vi "main.vi"() -> ()   [LabVIEW 2019]
panel:
  out "Position":i32
  in  "OK":bool
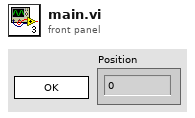
[diagram p1: front panel]
types:
  T1 = enum32{"Invalid", "Standard", "Closed", "Hidden", "Minimized", "Maximized"}
  T2 = enum32{"invalid app kind", "Development System", "Run Time System", "Student Edition", "Embedded LabVIEW", "Evaluation", "Custom"}
  T3 = cluster{"Core":cluster{"Current VI Reference":refnum<vi>, "Close Panel on Exit?":bool}, "Your Boolean data":bool, "Your string data":string}
  T4 = cluster{"Current VI Reference":refnum<vi>, "Close Panel on Exit?":bool}
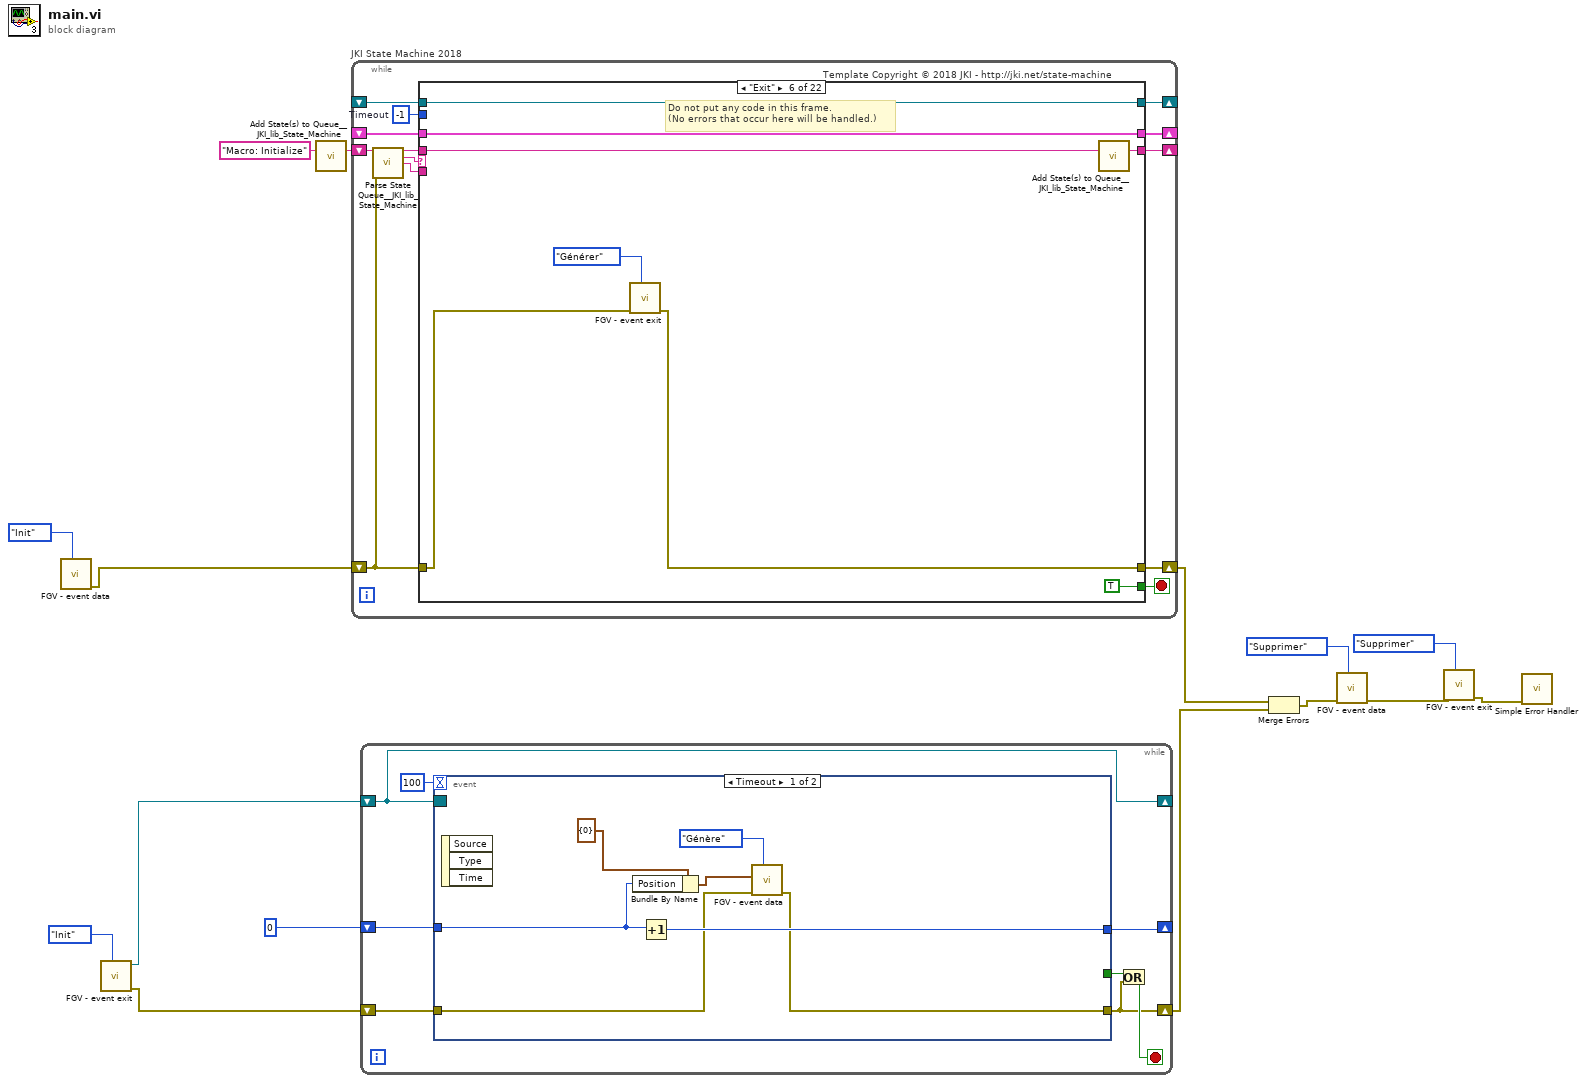
[diagram p0: block diagram]
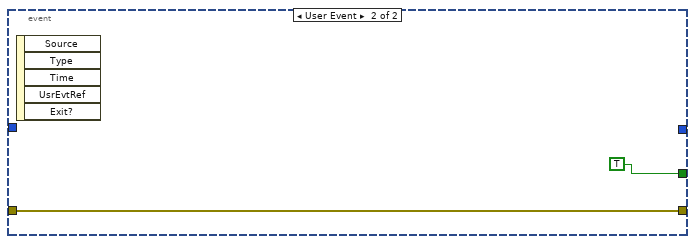
[diagram p2: hidden frame]
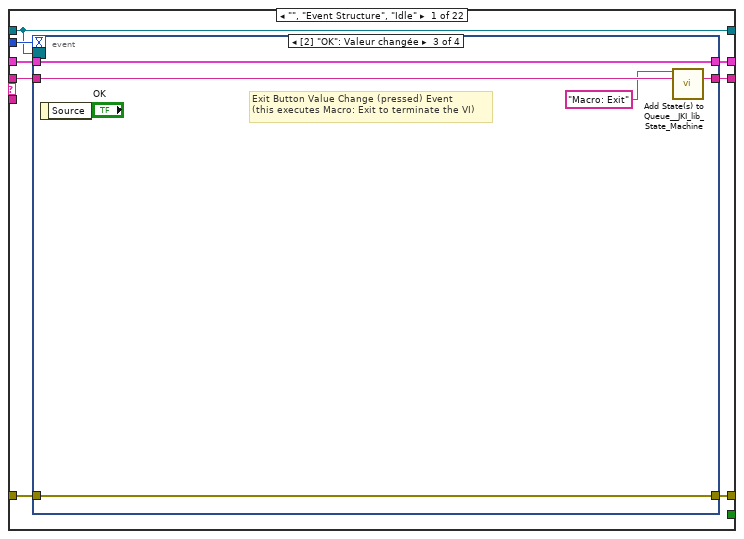
[diagram p3: hidden frame]
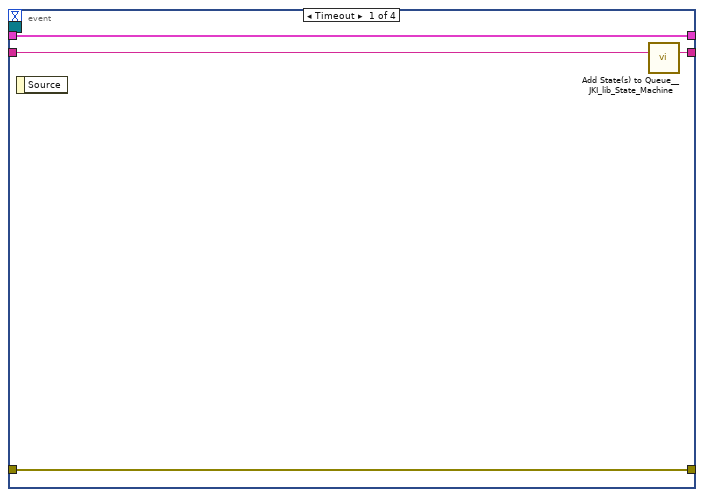
[diagram p4: hidden frame]
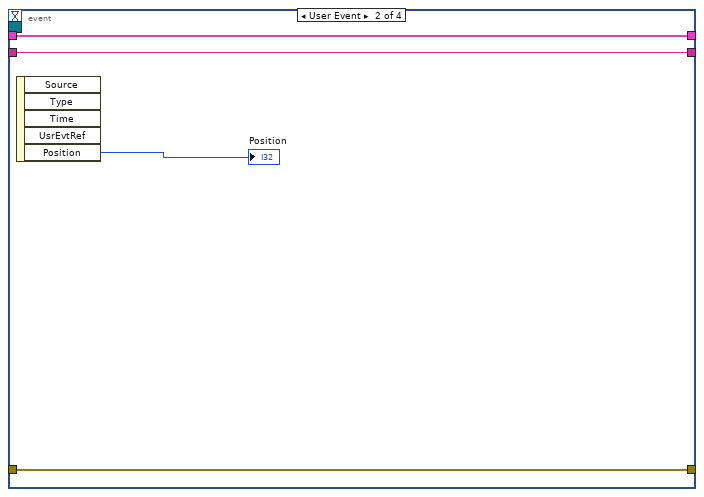
[diagram p5: hidden frame]
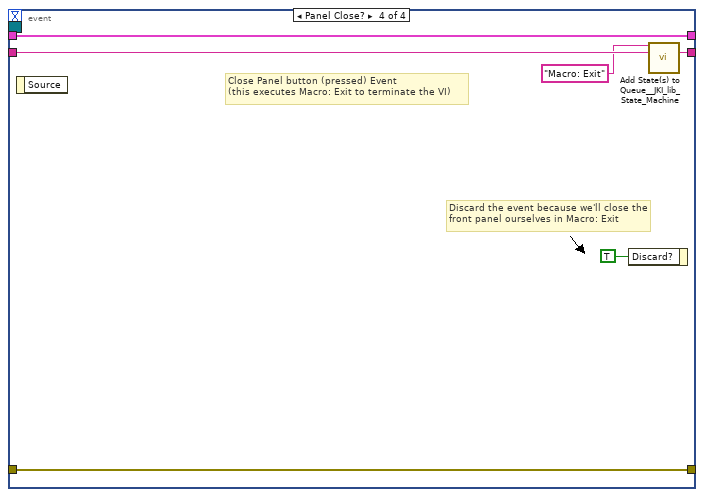
[diagram p6: hidden frame]
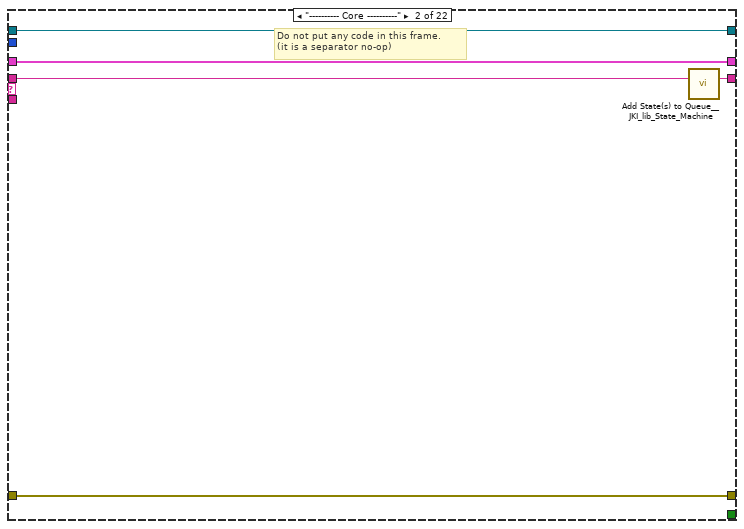
[diagram p7: hidden frame]
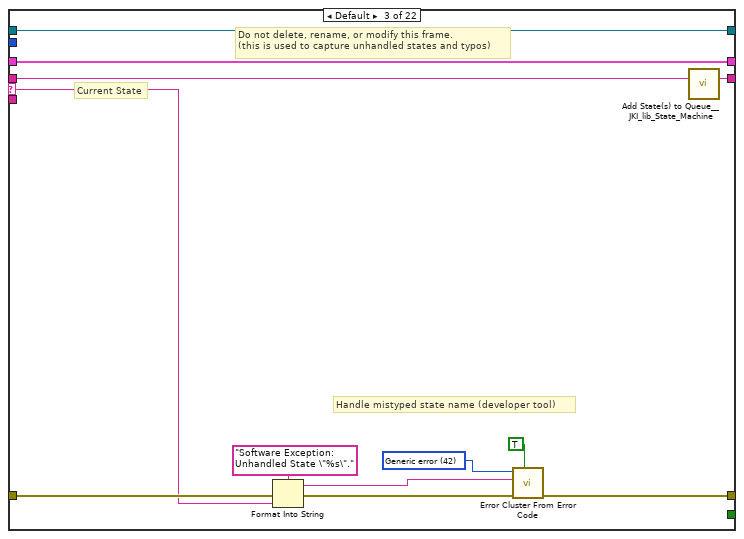
[diagram p8: hidden frame]
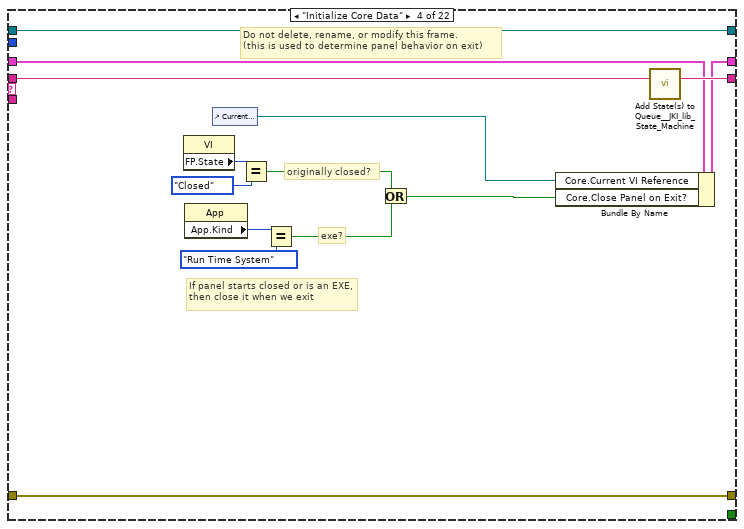
[diagram p9: hidden frame]
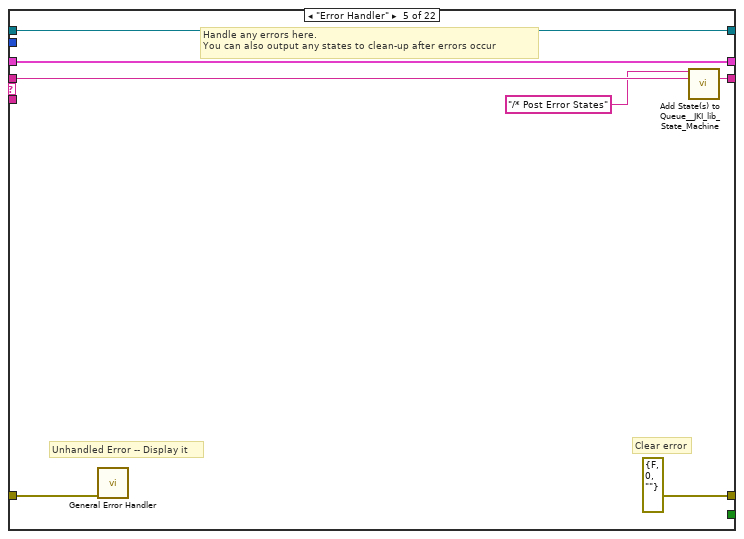
[diagram p10: hidden frame]
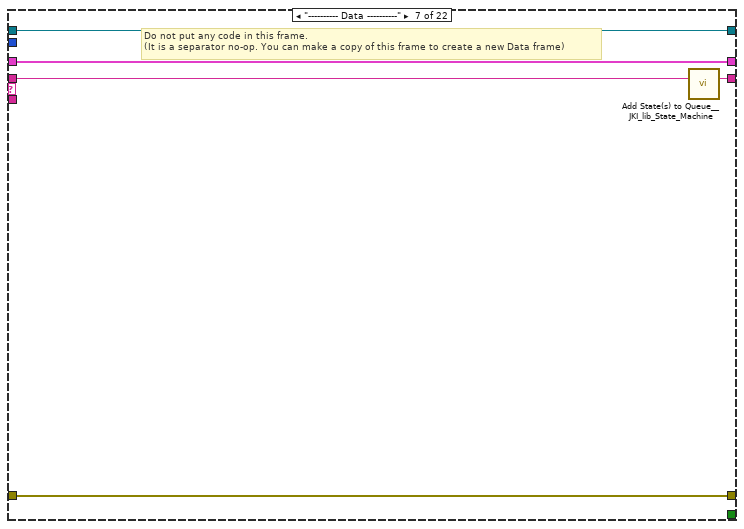
[diagram p11: hidden frame]
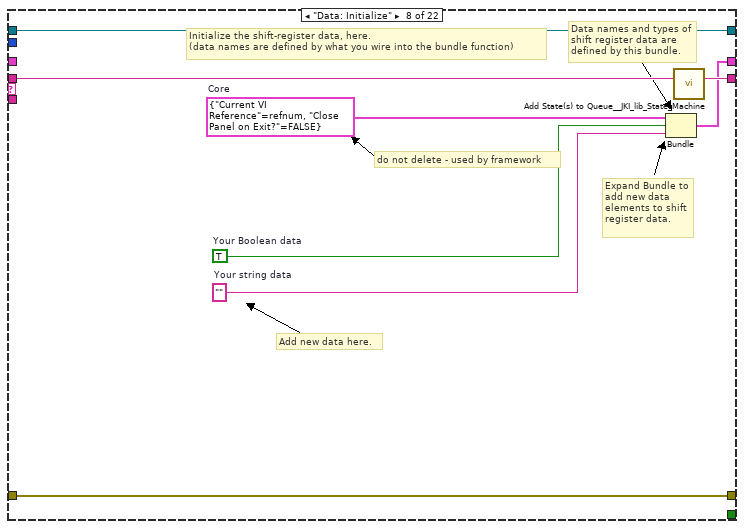
[diagram p12: hidden frame]
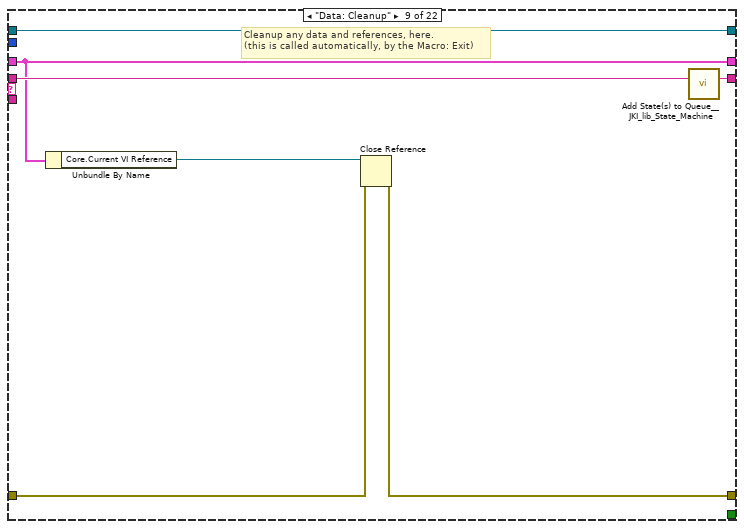
[diagram p13: hidden frame]
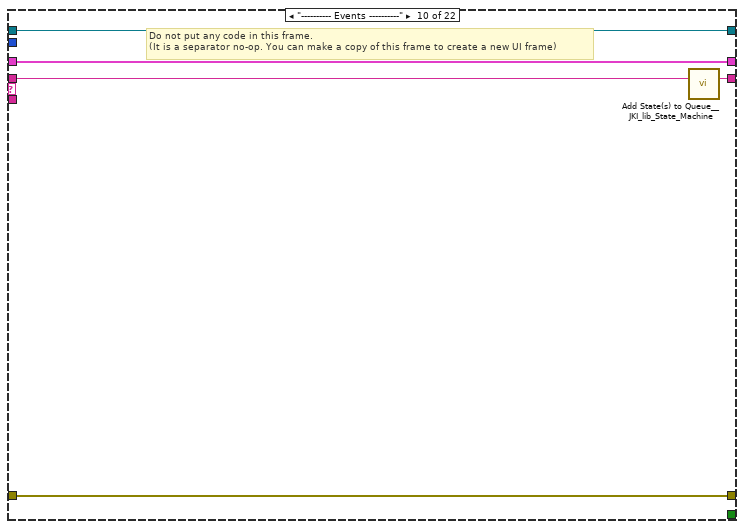
[diagram p14: hidden frame]
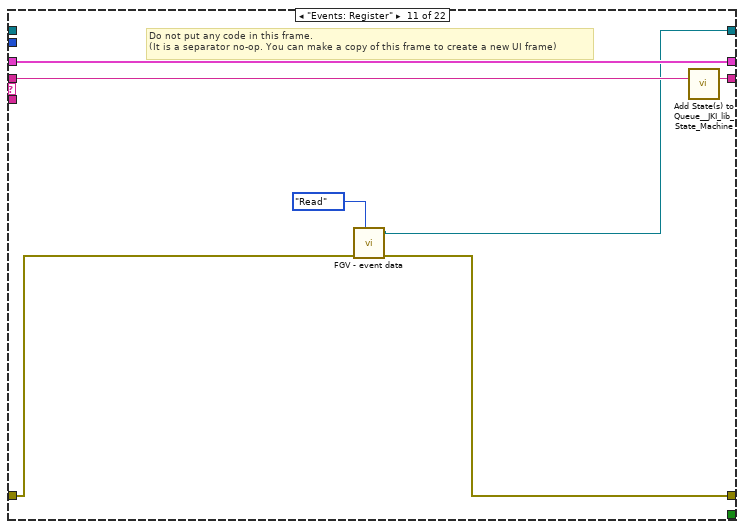
[diagram p15: hidden frame]
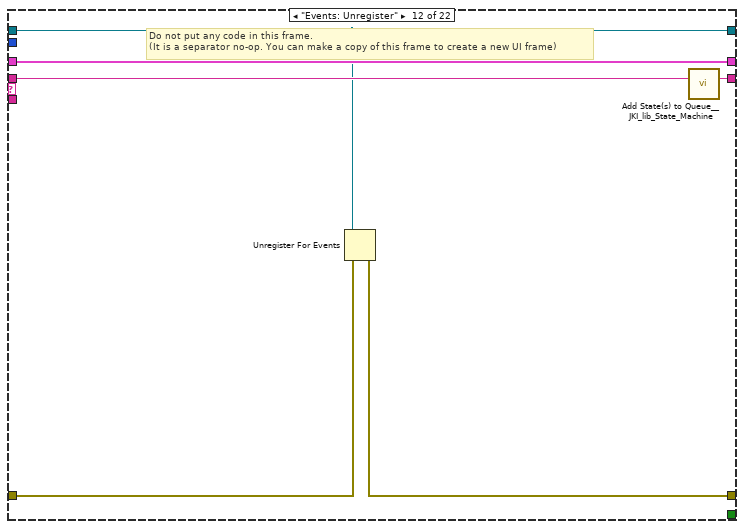
[diagram p16: hidden frame]
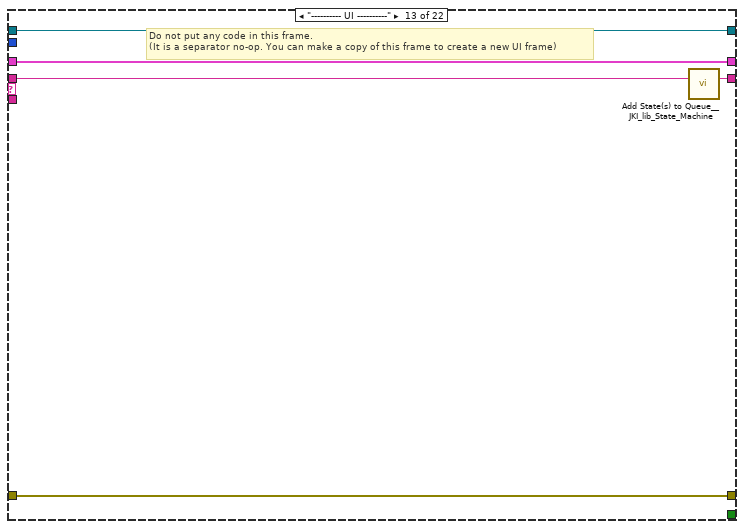
[diagram p17: hidden frame]
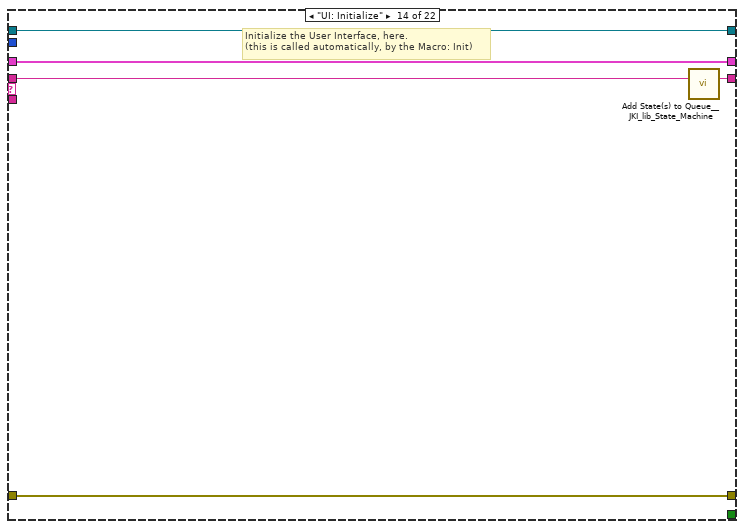
[diagram p18: hidden frame]
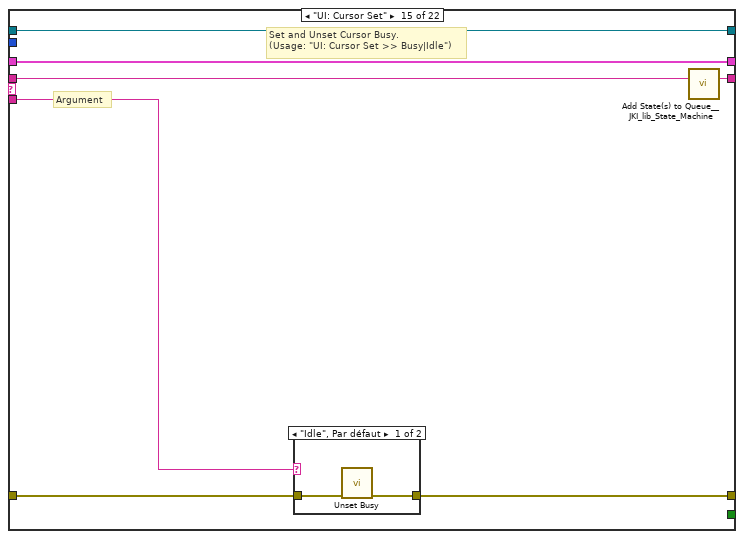
[diagram p19: hidden frame]
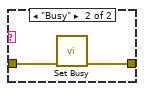
[diagram p20: hidden frame]
diagram:
  n1 = call "FGV - event data.vi"("Action (Read)"=enum16{"Init", "Read", "Génère", "Supprimer"}."Init") -> ("sortie d'erreur"=w13:errorcluster)  [unwired: 9 in, 1 out]
  n2 = call "FGV - event exit.vi"("Action (Read)"=enum16{"Init", "Read", "Générer", "Supprimer"}."Init") -> ("sortie d'erreur"=w6:errorcluster, "Refnum d'abonnement à des événements"=w11:refnum<event-registration>)  [unwired: 9 in]
  n3 = call <vilib>:"Add State(s) to Queue__JKI_lib_State_Machine.vi"("State(s) in (\"\")"="Macro: Initialize") -> ("States Out"=w15:string)  [unwired: 14 in]
  n4 = while "JKI State Machine 2018" {
    shift-right: [w21] -> _
    shift-left: _ -> [w20]
    shift-right: [w24] -> w9
    shift-left: w13 -> [w18]
    shift-right: [w23] -> _
    shift-left: w15 -> [w25]
    shift-right: [w17] -> _
    shift-left: _ -> [w16]
    stop <- w22 stop-if-true
    w19 = -1  # Timeout
    # "Template Copyright © 2018 JKI - http://jki.net/state-machine"
    n5 = call <vilib>:"Parse State Queue__JKI_lib_State_Machine.vi"("State Queue"=w25, "Error In (no error)"=w18) -> ("Remaining States"=w27:string, "Current State"=w28:string, "Arguments"=w26:string)  [unwired: 11 in]
    n6 = case shown="\"Exit\"" w28 {
      selector: w28 -> [_ _ w62 _ _ _ _ _ _ _ _ _ _ _ _ _ _ _ _ _ _ _]
      tunnel: w27 -> [w36 w60 w66 w86 w93 w101 w106 w114 w121 w126 w133 w139 w144 w149 w156 w168 w238 w244 w255 w260 w265 w270]
      tunnel: w26 -> [_ _ _ _ _ _ _ _ _ _ _ _ _ _ w151 w162 _ _ _ _ _ _]
      tunnel: w20 -> [w34 w57 w64 w79 w90 w99 w103 _ w116 w123 w131 w137 w141 w147 w154 w164 w235 w241 w252 w257 w262 w267]
      tunnel: [w33 w58 w68 w83 errorcluster {"status"=FALSE, "code"=0, "source"=""} ("error out") w95 w104 w111 w117 w124 w128 w134 w142 w146 w152 w165 w236 w242 w253 w258 w263 w268] -> w24
      tunnel: w18 -> [w32 w58 w67 w83 w89 w96 w104 w111 w118 w124 w129 w135 w142 w146 w153 w166 w236 w242 w253 w258 w263 w268]
      tunnel: [w35 w59 w65 w85 w92 w100 w105 w113 w120 w125 w132 w138 w143 w148 w155 w167 w237 w243 w254 w259 w264 w269] -> w23
      tunnel: [_ _ _ _ _ TRUE _ _ _ _ _ _ _ _ _ _ _ _ _ _ _ _] -> w22
      tunnel: [w31 w57 w64 w84 w90 w99 w103 w112 w116 w123 w131 w137 w141 w147 w154 w164 w235 w241 w252 w257 w262 w267] -> w21
      tunnel: w19 -> [w30 _ _ _ _ _ _ _ _ _ _ _ _ _ _ _ _ _ _ _ _ _]
      tunnel: [w29 w56 w61 w73 w87 w97 w102 w107 w115 w122 w130 w136 w140 w145 w150 w161 w234 w239 w245 w256 w261 w266] -> w17
      tunnel: w16 -> [w29 w56 w61 w73 w87 w97 w102 w107 w115 w122 _ w136 w140 w145 w150 w161 w234 w239 w245 w256 w261 w266]
      frame "", "Event Structure", "Idle" {
        n7 = event shown="[2] \"OK\": Valeur changée" {
          selector: w29 -> [_ _ _ _]
          dyn-events: _ -> [_ _ _ _]
          timeout: w30 -> [_ _ _ _]
          tunnel: w36 -> [w40 w42 w49 w55]
          tunnel: [w39 w42 w48 w54] -> w35
          tunnel: w34 -> [w37 w43 w46 w52]
          tunnel: [w38 w41 w47 w53] -> w33
          tunnel: w32 -> [w38 w41 w47 w53]
          tunnel: [w37 w43 w46 w52] -> w31
          event Timeout {
            n8 = event-data() -> ()  [unwired: 1 in, 1 out]
            n9 = call <vilib>:"Add State(s) to Queue__JKI_lib_State_Machine.vi"("State(s) in (\"\")"=w40) -> ("States Out"=w39:string)  [unwired: 14 in]
          }
          event User Event {
            n10 = event-data() -> ("Position"=→"Position":i32)  [unwired: 1 in, 4 out]
          }
          event "OK": Value Change {
            # "Exit Button Value Change (pressed) Event\n(this executes Macro: Exit to terminate the VI)"
            n11 = event-data() -> ()  [unwired: 1 in, 1 out]
            n12 = call <vilib>:"Add State(s) to Queue__JKI_lib_State_Machine.vi"("State(s) in Front (\"\")"="Macro: Exit", "State(s) in (\"\")"=w49) -> ("States Out"=w48:string)  [unwired: 13 in]
          }
          event Panel Close? {
            # "Discard the event because we'll close the front panel ourselves in Macro: Exit"
            # "Close Panel button (pressed) Event\n(this executes Macro: Exit to terminate the VI)"
            n13 = event-data() -> ()  [unwired: 1 in, 1 out]
            n14 = event-data("Discard?"=TRUE) -> ()  [unwired: 1 in, 1 out]
            n15 = call <vilib>:"Add State(s) to Queue__JKI_lib_State_Machine.vi"("State(s) in Front (\"\")"="Macro: Exit", "State(s) in (\"\")"=w55) -> ("States Out"=w54:string)  [unwired: 13 in]
          }
        }
      }
      frame "---------- Core ----------" {
        # "Do not put any code in this frame.\n(it is a separator no-op)"
        n16 = call <vilib>:"Add State(s) to Queue__JKI_lib_State_Machine.vi"("State(s) in (\"\")"=w60) -> ("States Out"=w59:string)  [unwired: 14 in]
      }
      frame Default {
        w71 = 42 items=["No error", "Argument error", "Memory is full", "Out of zone", "End of file", "File already open", "Generic file I/O error", "File not found", "File permission error", "Disk is full", "Duplicate path", "Too many files open", "System feature not enabled", "Resource file not found", "Cannot add resource", "Resource not found", "Image not found", "Image memory error", "Pen does not exist", "Config type invalid", "Config token not found", "Config parse error", "Config memory error", "Bad external code format", "Bad external code offset", "External code not present", "Null window", "Destroy window error", "Null menu", "Print aborted", "Bad print record", "Print driver error", "Windows error during printing", "Memory error during printing", "Print dialog error", "Generic print error", "Invalid device refnum", "Device not found", "Device parameter error", "Device unit error", "Cannot open device", "Device call aborted", "Generic error", "Cancelled by user", "Object ID too low", "Object ID too high", "Object not in heap", "Unknown heap", "Unknown object (invalid DefProc)", "Unknown object (DefProc not in table)", "Message out of range", "Invalid (null) method", "Unknown message", "Manager call not supported", "Bad address", "Network operation in progress", "Network operation timed out", "Connection is busy", "Network attribute not supported", "Network error", "Address in use", "System out of memory", "Connection aborted", "Connection refused", "Not connected", "Already connected", "Connection closed", "Initialization error (interapplication manager)", "Bad occurrence", "Wait on unbound occurrence handler", "Occurrence queue overflow", "Datalog type conflict", "Unused", "Unrecognized type (interapplication manager)", "Memory corrupt", "Failed to make temporary DLL", "Old CIN version", "Drag socket not found", "Failed to load drop-object", "Failed to register OLE object", "Failed to release OLE object", "Format specifier type mismatch", "Unknown format specifier", "Too few format specifiers", "Too many format specifiers", "Scan failed", "Newer CIN version", "Error converting to variant", "Runtime menu error", "Password tampered", "Variant attribute not found", "Incompatible variant data type", "Event data is not available", "Event Store is not present", "Occurrence is not found", "Event Queue is not created", "Event info is not available", "Refnum passed is NULL", "Error retrieving Class GUID", "Error retrieving CoClass GUID", "Error retrieving TypeLib GUID.", "Bad built application magic bytes.", "Specific driver is different from the specific driver associated with the Logical Name.", "There is no session opened to the class driver.", "Max Error", "MAX - Error with config objects", "MAX - Error loading configuration", "MAX - Group not supported"]
        # "Current State"
        # "Do not delete, rename, or modify this frame.\n(this is used to capture unhandled states and typos)"
        # "Handle mistyped state name (developer tool)"
        n17 = Format Into String(format string="Software Exception: Unhandled State \"%s\"." ("message"), error in=w67, w62) -> (resulting string=w70:string, error out=w69:errorcluster)  [unwired: 1 in]
        n18 = call <vilib>:"Error Cluster From Error Code.vi"("show call chain? (False)"=TRUE, "error in (no error)"=w69, "error message (\"\")"=w70, "error code (0)"=w71) -> ("error out"=w68:errorcluster)  [unwired: 5 in]
        n19 = call <vilib>:"Add State(s) to Queue__JKI_lib_State_Machine.vi"("State(s) in (\"\")"=w66) -> ("States Out"=w65:string)  [unwired: 14 in]
      }
      frame "Initialize Core Data" {
        # "Do not delete, rename, or modify this frame.\n(this is used to determine panel behavior on exit)"
        # "originally closed?"
        # "exe?"
        # "If panel starts closed or is an EXE, then close it when we exit"
        n20 = property class="VI"() -> ("FP.State"=w76:T1)  [unwired: 2 in, 2 out]
        n21 = property class="App"() -> ("App.Kind"=w82:T2)  [unwired: 2 in, 2 out]
        n22 = control-ref of="Current VI Reference"() -> (w77:refnum<vi>)
        n23 = Equal?(x=w76, y=T1."Closed" ("Front Panel Window:State")) -> (x = y?=w74:bool)
        n24 = Equal?(x=w82, y=T2."Run Time System" ("Application:Kind")) -> (x = y?=w80:bool)
        n25 = Or(x=w74, y=w80) -> (x .or. y?=w78:bool)
        n26 = Bundle By Name(cluster=w79, "Core.Current VI Reference"=w77, "Core.Close Panel on Exit?"=w78) -> (w84:T3)
        n27 = call <vilib>:"Add State(s) to Queue__JKI_lib_State_Machine.vi"("State(s) in (\"\")"=w86) -> ("States Out"=w85:string)  [unwired: 14 in]
      }
      frame "Error Handler" {
        # "Unhandled Error -- Display it"
        # "Handle any errors here.\nYou can also output any states to clean-up after errors occur"
        # "Clear error"
        n28 = call <vilib>:"General Error Handler.vi"("error in (no error)"=w89) -> ()  [unwired: 10 in, 5 out]
        n29 = call <vilib>:"Add State(s) to Queue__JKI_lib_State_Machine.vi"("State(s) in Front (\"\")"="/* Post Error States", "State(s) in (\"\")"=w93) -> ("States Out"=w92:string)  [unwired: 13 in]
      }
      frame "Exit" {
        # "Do not put any code in this frame.\n(No errors that occur here will be handled.)"
        n30 = call "FGV - event exit.vi"("Action (Read)"=enum16{"Init", "Read", "Générer", "Supprimer"}."Générer", "entrée d'erreur (pas d'erreur)"=w96) -> ("sortie d'erreur"=w95:errorcluster)  [unwired: 8 in, 1 out]
        n31 = call <vilib>:"Add State(s) to Queue__JKI_lib_State_Machine.vi"("State(s) in (\"\")"=w101) -> ("States Out"=w100:string)  [unwired: 14 in]
      }
      frame "---------- Data ----------" {
        # "Do not put any code in this frame.\n(It is a separator no-op. You can make a copy of this frame to create a new Data frame)"
        n32 = call <vilib>:"Add State(s) to Queue__JKI_lib_State_Machine.vi"("State(s) in (\"\")"=w106) -> ("States Out"=w105:string)  [unwired: 14 in]
      }
      frame "Data: Initialize" {
        w108 = T4 {"Current VI Reference"=refnum, "Close Panel on Exit?"=FALSE}  # Core
        w110 = TRUE  # Your Boolean data
        w109 = ""  # Your string data
        # "do not delete - used by framework"
        # "Expand Bundle to add new data elements to shift register data."
        # "Add new data here."
        # "Data names and types of shift register data are defined by this bundle."
        # "Initialize the shift-register data, here.\n(data names are defined by what you wire into the bundle function)"
        n33 = Bundle("Core"=w108, "Your Boolean data"=w110, "Your string data"=w109) -> (w112:T3)  [unwired: 1 in]
        n34 = call <vilib>:"Add State(s) to Queue__JKI_lib_State_Machine.vi"("State(s) in (\"\")"=w114) -> ("States Out"=w113:string)  [unwired: 14 in]
      }
      frame "Data: Cleanup" {
        # "Cleanup any data and references, here.\n(this is called automatically, by the Macro: Exit)"
        n35 = Unbundle By Name(w116) -> ("Core.Current VI Reference"=w119:refnum<vi>)
        n36 = Close Reference(reference=w119, error in (no error)=w118) -> (error out=w117:errorcluster)
        n37 = call <vilib>:"Add State(s) to Queue__JKI_lib_State_Machine.vi"("State(s) in (\"\")"=w121) -> ("States Out"=w120:string)  [unwired: 14 in]
      }
      frame "---------- Events ----------" {
        # "Do not put any code in this frame.\n(It is a separator no-op. You can make a copy of this frame to create a new UI frame)"
        n38 = call <vilib>:"Add State(s) to Queue__JKI_lib_State_Machine.vi"("State(s) in (\"\")"=w126) -> ("States Out"=w125:string)  [unwired: 14 in]
      }
      frame "Events: Register" {
        # "Do not put any code in this frame.\n(It is a separator no-op. You can make a copy of this frame to create a new UI frame)"
        n39 = call "FGV - event data.vi"("Action (Read)"=enum16{"Init", "Read", "Génère", "Supprimer"}."Read", "entrée d'erreur (pas d'erreur)"=w129) -> ("sortie d'erreur"=w128:errorcluster, "Refnum d'abonnement à des événements"=w130:refnum<event-registration>)  [unwired: 8 in]
        n40 = call <vilib>:"Add State(s) to Queue__JKI_lib_State_Machine.vi"("State(s) in (\"\")"=w133) -> ("States Out"=w132:string)  [unwired: 14 in]
      }
      frame "Events: Unregister" {
        # "Do not put any code in this frame.\n(It is a separator no-op. You can make a copy of this frame to create a new UI frame)"
        n41 = Unregister For Events(event registration refnum=w136, error in=w135) -> (error out=w134:errorcluster)
        n42 = call <vilib>:"Add State(s) to Queue__JKI_lib_State_Machine.vi"("State(s) in (\"\")"=w139) -> ("States Out"=w138:string)  [unwired: 14 in]
      }
      frame "---------- UI ----------" {
        # "Do not put any code in this frame.\n(It is a separator no-op. You can make a copy of this frame to create a new UI frame)"
        n43 = call <vilib>:"Add State(s) to Queue__JKI_lib_State_Machine.vi"("State(s) in (\"\")"=w144) -> ("States Out"=w143:string)  [unwired: 14 in]
      }
      frame "UI: Initialize" {
        # "Initialize the User Interface, here.\n(this is called automatically, by the Macro: Init)"
        n44 = call <vilib>:"Add State(s) to Queue__JKI_lib_State_Machine.vi"("State(s) in (\"\")"=w149) -> ("States Out"=w148:string)  [unwired: 14 in]
      }
      frame "UI: Cursor Set" {
        # "Argument"
        # "Set and Unset Cursor Busy.\n(Usage: \"UI: Cursor Set >> Busy|Idle\")"
        n45 = case shown="\"Idle\", Par défaut" w151 {
          tunnel: w153 -> [w158 w160]
          tunnel: [w157 w159] -> w152
          frame "Idle", Default {
            n46 = call <vilib>:"Unset Busy.vi"("error in (no error)"=w158) -> ("error out"=w157:errorcluster)  [unwired: 10 in]
          }
          frame "Busy" {
            n47 = call <vilib>:"Set Busy.vi"("error in (no error)"=w160) -> ("error out"=w159:errorcluster)  [unwired: 9 in, 1 out]
          }
        }
        n48 = call <vilib>:"Add State(s) to Queue__JKI_lib_State_Machine.vi"("State(s) in (\"\")"=w156) -> ("States Out"=w155:string)  [unwired: 14 in]
      }
      frame "UI: Front Panel State" {
        # "Argument"
        # "Set Front Panel Open or Closed\n(Usage: \"UI: Front Panel State >> Open|Close\")"
        n49 = Unbundle By Name(w164) -> ("Core.Current VI Reference"=w163:refnum<vi>)
        n50 = case shown="\"Minimize\", \"Minimized\"" w162 {
          tunnel: w166 -> [w174 w189 w200 w213 w226]
          tunnel: [w176 w190 w202 w215 w228] -> w165
          tunnel: w163 -> [w175 w187 w201 w214 w227]
          frame "Open", "Standard", Default {
            w169 = T1."Standard" ("State")
            n51 = property class="VI"(reference=w175, error in=w174) -> (reference out=w172:refnum<vi>, error out=w173:errorcluster, "FP.State"=w171:T1)
            n52 = Not Equal?(x=w171, y=w169) -> (x != y?=w170:bool)
            n53 = case shown="Vrai" w170 {
              tunnel: [w180 w182] -> w176
              tunnel: w173 -> [w179 w182]
              tunnel: w172 -> [w178 _]
              tunnel: w169 -> [w177 _]
              frame True {
                n54 = invoke class="VI" method="FA.Ouvrir"(reference=w178, error in=w179, "Activate"=TRUE, "State"=w177) -> (error out=w180:errorcluster)  [unwired: 1 in, 4 out]
              }
              frame False {
              }
            }
          }
          frame "Close", "Closed" {
            n55 = property class="VI"(reference=w187, error in=w189) -> (reference out=w186:refnum<vi>, error out=w188:errorcluster, "FP.State"=w184:T1)
            n56 = Not Equal?(x=w184, y=T1."Closed" ("Front Panel Window:State")) -> (x != y?=w183:bool)
            n57 = case shown="Vrai" w183 {
              tunnel: [w191 w194] -> w190
              tunnel: w188 -> [w191 w193]
              tunnel: w186 -> [_ w192]
              frame False {
              }
              frame True {
                n58 = invoke class="VI" method="FA.Fermer"(reference=w192, error in=w193) -> (error out=w194:errorcluster)  [unwired: 1 in, 2 out]
              }
            }
          }
          frame "Hidden", "Hide" {
            w195 = T1."Hidden" ("State")
            n59 = property class="VI"(reference=w201, error in=w200) -> (reference out=w198:refnum<vi>, error out=w199:errorcluster, "FP.State"=w197:T1)
            n60 = Not Equal?(x=w197, y=w195) -> (x != y?=w196:bool)
            n61 = case shown="Vrai" w196 {
              tunnel: [w206 w207] -> w202
              tunnel: w199 -> [w205 w207]
              tunnel: w198 -> [w204 _]
              tunnel: w195 -> [w203 _]
              frame True {
                n62 = invoke class="VI" method="FA.Ouvrir"(reference=w204, error in=w205, "State"=w203) -> (error out=w206:errorcluster)  [unwired: 2 in, 4 out]
              }
              frame False {
              }
            }
          }
          frame "Minimize", "Minimized" {
            w208 = T1."Minimized" ("State")
            n63 = property class="VI"(reference=w214, error in=w213) -> (reference out=w211:refnum<vi>, error out=w212:errorcluster, "FP.State"=w210:T1)
            n64 = Not Equal?(x=w210, y=w208) -> (x != y?=w209:bool)
            n65 = case shown="Vrai" w209 {
              tunnel: [w219 w220] -> w215
              tunnel: w212 -> [w218 w220]
              tunnel: w211 -> [w217 _]
              tunnel: w208 -> [w216 _]
              frame True {
                n66 = invoke class="VI" method="FA.Ouvrir"(reference=w217, error in=w218, "State"=w216) -> (error out=w219:errorcluster)  [unwired: 2 in, 4 out]
              }
              frame False {
              }
            }
          }
          frame "Maximize", "Maximized" {
            w221 = T1."Maximized" ("State")
            n67 = property class="VI"(reference=w227, error in=w226) -> (reference out=w224:refnum<vi>, error out=w225:errorcluster, "FP.State"=w223:T1)
            n68 = Not Equal?(x=w223, y=w221) -> (x != y?=w222:bool)
            n69 = case shown="Vrai" w222 {
              tunnel: [w232 w233] -> w228
              tunnel: w225 -> [w231 w233]
              tunnel: w224 -> [w230 _]
              tunnel: w221 -> [w229 _]
              frame True {
                n70 = invoke class="VI" method="FA.Ouvrir"(reference=w230, error in=w231, "State"=w229) -> (error out=w232:errorcluster)  [unwired: 2 in, 4 out]
              }
              frame False {
              }
            }
          }
        }
        n71 = call <vilib>:"Add State(s) to Queue__JKI_lib_State_Machine.vi"("State(s) in (\"\")"=w168) -> ("States Out"=w167:string)  [unwired: 14 in]
      }
      frame "---------- Macro ----------" {
        # "Do not put any code in this frame.\n(It is a separator no-op. You can make a copy of this frame to create a new Macro frame)"
        n72 = call <vilib>:"Add State(s) to Queue__JKI_lib_State_Machine.vi"("State(s) in (\"\")"=w238) -> ("States Out"=w237:string)  [unwired: 14 in]
      }
      frame "Macro: Initialize" {
        # "Initialization Macro\n(This is called once, when the VI starts)"
        n73 = call <vilib>:"Add State(s) to Queue__JKI_lib_State_Machine.vi"("State(s) in Front (\"\")"="Data: Initialize\nInitialize Core Data\nEvents: Register\nUI: Initialize\nUI: Front Panel State >> Open", "State(s) in (\"\")"=w244) -> ("States Out"=w243:string)  [unwired: 13 in]
      }
      frame "Macro: Exit" {
        # "Exit Macro\n(This is called once, when the VI exits)"
        n74 = Unbundle By Name(w252) -> ("Core.Close Panel on Exit?"=w251:bool)
        n75 = Select(t="UI: Front Panel State >> Close", s=w251, f="") -> (s? t:f=w248:string)
        n76 = call <vilib>:"Add State(s) to Queue__JKI_lib_State_Machine.vi"("State(s) in (\"\")"=w248, "State(s) at Back (\"\")"="Data: Cleanup\nEvents: Unregister\nExit") -> ("States Out"=w246:string)  [unwired: 13 in]
        n77 = call <vilib>:"Add State(s) to Queue__JKI_lib_State_Machine.vi"("State(s) in Front (\"\")"=w246, "State(s) in (\"\")"=w255) -> ("States Out"=w254:string)  [unwired: 13 in]
      }
      frame "---------- New Category ----------" {
        # "Template Separator\n(You can make a copy of, or modify, this frame)"
        n78 = call <vilib>:"Add State(s) to Queue__JKI_lib_State_Machine.vi"("State(s) in (\"\")"=w260) -> ("States Out"=w259:string)  [unwired: 14 in]
      }
      frame "New Category: 1" {
        # "Your code here.\n(You can make a copy of, or modify, this frame)"
        n79 = call <vilib>:"Add State(s) to Queue__JKI_lib_State_Machine.vi"("State(s) in (\"\")"=w265) -> ("States Out"=w264:string)  [unwired: 14 in]
      }
      frame "New Category: 2" {
        # "Your code here.\n(You can make a copy of, or modify, this frame)"
        n80 = call <vilib>:"Add State(s) to Queue__JKI_lib_State_Machine.vi"("State(s) in (\"\")"=w270) -> ("States Out"=w269:string)  [unwired: 14 in]
      }
    }
  }
  n81 = while {
    shift-right: [w276] -> _
    shift-left: 0 -> [w277]
    shift-right: [w274] -> _
    shift-left: w11 -> [w274]
    shift-right: [w271] -> w5
    shift-left: w6 -> [w272]
    stop <- w275 stop-if-true
    n82 = event shown="[0] Timeout" {
      selector: w274 -> [_ _]
      dyn-events: _ -> [_ _]
      timeout: 100 -> [_ _]
      tunnel: w277 -> [w284 _]
      tunnel: [w285 _] -> w276
      tunnel: [_ TRUE] -> w273
      tunnel: [w280 w286] -> w271
      tunnel: w272 -> [w279 w286]
      event Timeout {
        n83 = event-data() -> ()  [unwired: 1 in, 3 out]
        n84 = Bundle By Name(cluster=cluster{"Position":i32} {"Position"=0} ("données d'événement"), "Position"=w284) -> (w281:cluster{"Position":i32})
        n85 = Increment(x=w284) -> (x+1=w285:i32)
        n86 = call "FGV - event data.vi"("Action (Read)"=enum16{"Init", "Read", "Génère", "Supprimer"}."Génère", "entrée d'erreur (pas d'erreur)"=w279, "Event Data"=w281) -> ("sortie d'erreur"=w280:errorcluster)  [unwired: 7 in, 1 out]
      }
      event User Event {
        n87 = event-data() -> ()  [unwired: 1 in, 5 out]
      }
    }
    n88 = Or(x=w273, y=w271) -> (x .or. y?=w275:bool)
  }
  n89 = Merge Errors(w9, w5) -> (w8:errorcluster)
  n90 = call "FGV - event data.vi"("Action (Read)"=enum16{"Init", "Read", "Génère", "Supprimer"}."Supprimer", "entrée d'erreur (pas d'erreur)"=w8) -> ("sortie d'erreur"=w7:errorcluster)  [unwired: 8 in, 1 out]
  n91 = call "FGV - event exit.vi"("Action (Read)"=enum16{"Init", "Read", "Générer", "Supprimer"}."Supprimer", "entrée d'erreur (pas d'erreur)"=w7) -> ("sortie d'erreur"=w10:errorcluster)  [unwired: 8 in, 1 out]
  n92 = call <vilib>:"Simple Error Handler.vi"("error in (no error)"=w10) -> ()  [unwired: 4 in, 5 out]
